vi "Nested Active Status.vi"(8 "error in (no error)":errorcluster, 11 "Module in":refnum<class "Module.lvclass">) -> (0 "error out":errorcluster, 1 "Inactive Nested":T3(array[cluster]), 2 "Active Nested":T3(array[cluster]), 3 "Module out":refnum<class "Module.lvclass">)   [LabVIEW 2020, in "Volatus.lvlib" / "Module.lvclass"]
uses:
  Module.lvclass
  Module.lvclass/Module.ctl
  MessageQ/MessageQ.lvclass
  State.ctl
  Module Status.ctl
  Volatus.lvlib
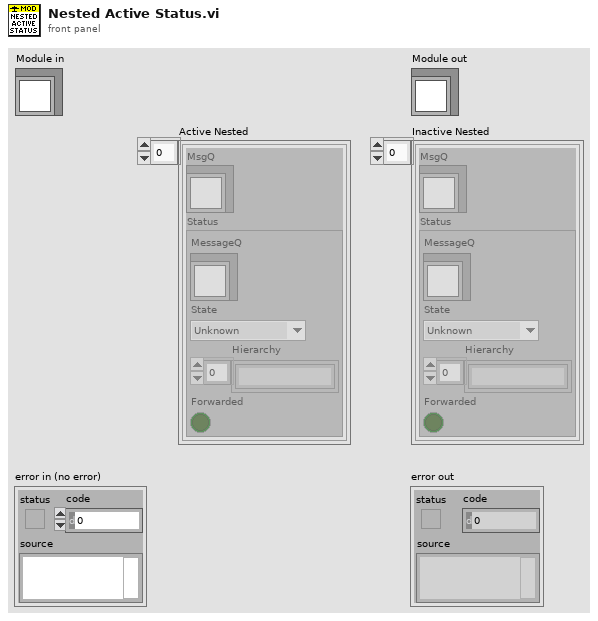
[diagram p1: front panel]
types:
  T1 = typedef "Volatus.lvlib/Module Status.ctl" = cluster{"MessageQ":refnum<class "MessageQ.lvclass">, "State":T2, "Hierarchy":string[], "Forwarded":bool}
  T2 = typedef "Volatus.lvlib/Module.lvclass/State.ctl" = enum16{"Unknown", "Launched", "Starting", "Running", "Stopping", "Stopped", "Error - Starting", "Error - Run", "Error - Stopping"}
  T3 = cluster{"MsgQ":refnum<class "MessageQ.lvclass">, "Status":T1}[]
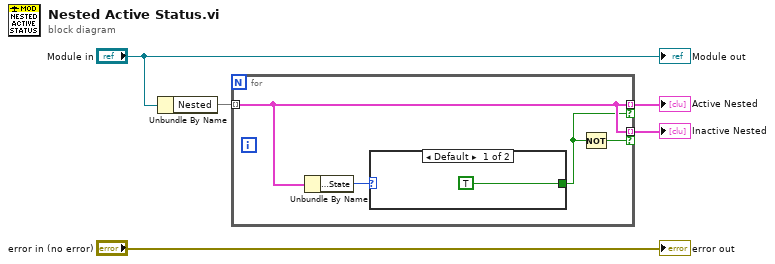
[diagram p0: block diagram]
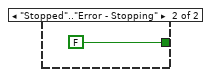
[diagram p2: hidden frame]
diagram:
  n1 = Unbundle By Name("Module in") -> ("Nested"=w4:map{refnum<class "MessageQ.lvclass">, T1})
  n2 = for {
    tunnel: w4 -> [w8] mode=indexing
    tunnel: [w8] -> w2 mode=indexing if=w7
    tunnel: [w8] -> w1 mode=indexing if=w6
    n3 = Unbundle By Name(w8) -> ("Status.State"=w9:T2)
    n4 = case shown="Default" w9 {
      tunnel: [TRUE FALSE] -> w7
      frame Default {
      }
      frame "Stopped".."Error - Stopping" {
      }
    }
    n5 = Not(x=w7) -> (.not. x?=w6:bool)
  }
  "Active Nested" <- w2
  "Inactive Nested" <- w1
  "error out" <- "error in (no error)"
  "Module out" <- "Module in"
